vi "Measurement Parser.vi"(8 "error in (no error)":errorcluster, 9 "Universal Power Meter.lvlib:Universal Card.lvclass":refnum<class "Universal Card.lvclass">, 10 "Data Array":dbl[](array[numeric]), 11 "Yokogawa WT1600 in":refnum<class "Yokogawa WT1600.lvclass">) -> (0 "error out":errorcluster, 2 "Waveform Graph":dynamicdata(graph), 3 "Yokogawa WT1600 out":refnum<class "Yokogawa WT1600.lvclass">)   [LabVIEW 2013, in "Universal Power Meter.lvlib" / "Yokogawa WT1600.lvlib" / "Yokogawa WT1600.lvclass"]
uses:
  Yokogawa WT1600.lvclass
  Universal Card Class/Universal Card.lvclass
  Measured Value Header Control.ctl
  Generic Instrument/Generic Card/Generic Card.lvclass/Generic Card.ctl
  Generic Instrument/Generic Card/Generic Card.lvclass
  Data Logger/Data Logger.lvclass
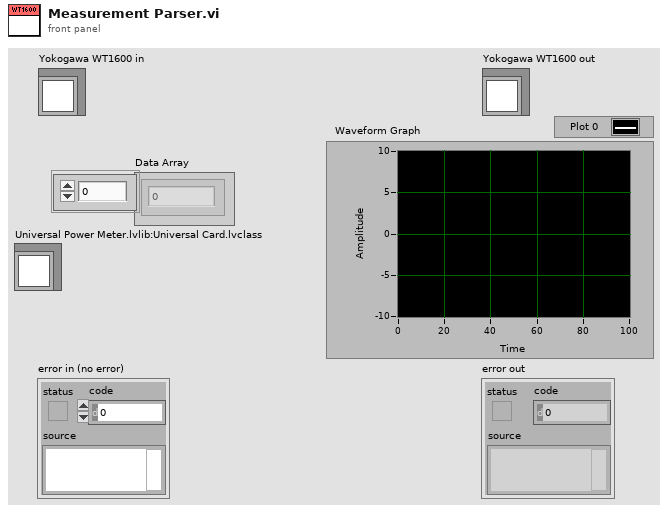
[diagram p1: front panel]
types:
  T1 = typedef "Measured Value Header Control.ctl" = enum16{"Current THD (%)", "Voltage THD (%)", "Amp-Hours", "Energy (Watt-hours)", "Frequency (Herts)", "Power (watts)", "Current RMS (amps)", "Voltage RMS (volts)"}
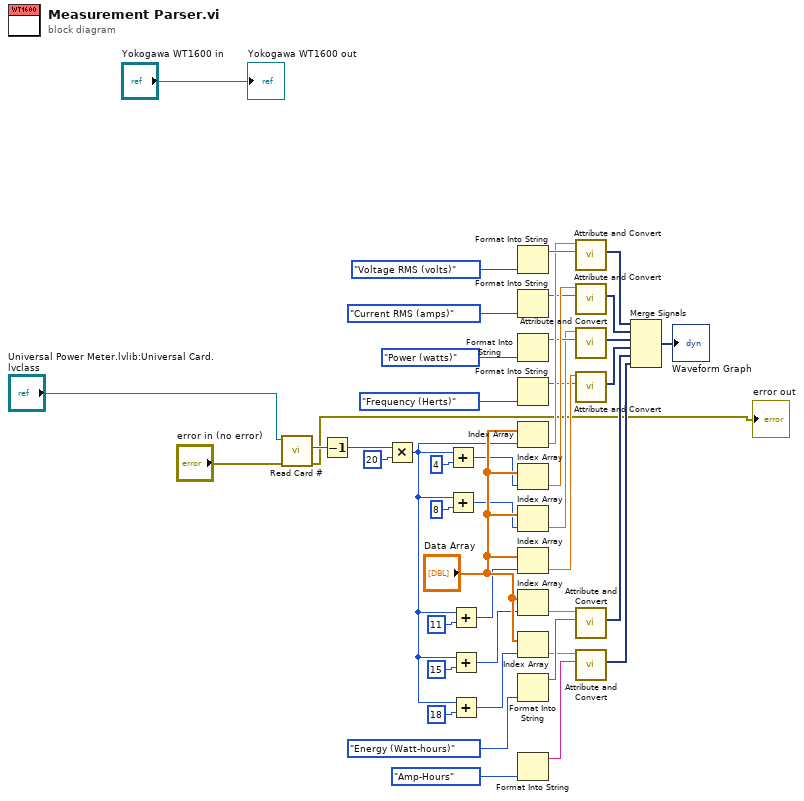
[diagram p0: block diagram]
diagram:
  n1 = call "Read Card #.vi"("error in (no error)"="error in (no error)", "Generic Card in"="Universal Power Meter.lvlib:Universal Card.lvclass") -> ("error out"=→"error out":errorcluster, "Card #"=w41:u8)  [unwired: 7 in, 1 out]
  n2 = Decrement(x=w41) -> (x-1=w38:u8)
  n3 = Multiply(x=w38, y=u8 20) -> (x*y=w10:u8)
  n4 = Add(x=w10, y=u8 4) -> (x+y=w15:u8)
  n5 = Add(x=w10, y=u8 8) -> (x+y=w9:u8)
  n6 = Add(x=w10, y=u8 11) -> (x+y=w8:u8)
  n7 = Add(x=w10, y=u8 15) -> (x+y=w7:u8)
  n8 = Add(x=w10, y=u8 18) -> (x+y=w6:u8)
  n9 = Format Into String(Measured_Value_Header_Control."Voltage RMS (volts)" ("Strings")) -> (resulting string=w40:string)  [unwired: 3 in, 1 out]
  n10 = Format Into String(Measured_Value_Header_Control."Current RMS (amps)" ("Strings")) -> (resulting string=w32:string)  [unwired: 3 in, 1 out]
  n11 = Format Into String(Measured_Value_Header_Control."Power (watts)" ("Strings")) -> (resulting string=w31:string)  [unwired: 3 in, 1 out]
  n12 = Format Into String(Measured_Value_Header_Control."Frequency (Herts)" ("Strings")) -> (resulting string=w26:string)  [unwired: 3 in, 1 out]
  n13 = Index Array(array="Data Array", index=w10) -> (element=w36:dbl)
  n14 = Index Array(array="Data Array", index=w15) -> (element=w34:dbl)
  n15 = Index Array(array="Data Array", index=w9) -> (element=w29:dbl)
  n16 = Index Array(array="Data Array", index=w8) -> (element=w28:dbl)
  n17 = Index Array(array="Data Array", index=w7) -> (element=w23:dbl)
  n18 = Index Array(array="Data Array", index=w6) -> (element=w20:dbl)
  n19 = Format Into String(Measured_Value_Header_Control."Energy (Watt-hours)" ("Strings")) -> (resulting string=w25:string)  [unwired: 3 in, 1 out]
  n20 = Format Into String(Measured_Value_Header_Control."Amp-Hours" ("Strings")) -> (resulting string=w18:string)  [unwired: 3 in, 1 out]
  n21 = call "Attribute and Convert.vi"("Signal Name"=w40, "Number in"=w36) -> ("Dynamic Signal Out"=w22:dynamicdata)  [unwired: 9 in]
  n22 = call "Attribute and Convert.vi"("Signal Name"=w32, "Number in"=w34) -> ("Dynamic Signal Out"=w21:dynamicdata)  [unwired: 9 in]
  n23 = call "Attribute and Convert.vi"("Signal Name"=w31, "Number in"=w29) -> ("Dynamic Signal Out"=w5:dynamicdata)  [unwired: 9 in]
  n24 = call "Attribute and Convert.vi"("Signal Name"=w26, "Number in"=w28) -> ("Dynamic Signal Out"=w4:dynamicdata)  [unwired: 9 in]
  n25 = call "Attribute and Convert.vi"("Signal Name"=w25, "Number in"=w23) -> ("Dynamic Signal Out"=w3:dynamicdata)  [unwired: 9 in]
  n26 = call "Attribute and Convert.vi"("Signal Name"=w18, "Number in"=w20) -> ("Dynamic Signal Out"=w2:dynamicdata)  [unwired: 9 in]
  n27 = Merge Signals(w22, w21, w5, w4, w3, w2) -> (→"Waveform Graph":dynamicdata)
  "Yokogawa WT1600 out" <- "Yokogawa WT1600 in"
